vi "NavX Variable Get.vi"(8 "error in":errorcluster) -> ()   [LabVIEW 2017]
uses:
  <vilib>/Rock Robotics/SystemInterfaces/spilib/spi_bus.ctl
  navx-mxp/labview/navX Library v2/IO/Open/Z900_navX_Open_SPI.vi
  navx-mxp/labview/navX Library v2/navX Library v2.lvlib
panel:
  in  "G Force":dbl=3.0
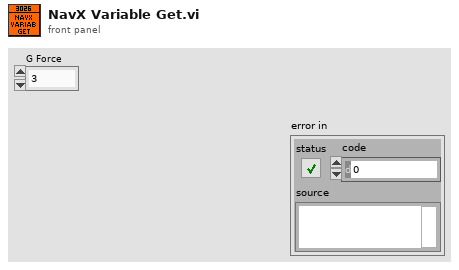
[diagram p1: front panel]
types:
  T1 = typedef "spi_bus.ctl" = enum16{"SPI On-Board, CS0", "SPI On-Board, CS1", "SPI On-Board, CS2", "SPI On-Board, CS3", "SPI MXP", "Invalid"}
  T2 = typedef "navX Library v2.lvlib/Z900_navX_DeviceTypeDef.ctl" = cluster{"Interface":cluster{"Protocol":T3, "Update Rate (4Hz-100Hz)":u8, "navX Open TypeDef":variant}, "Notify Packet":refnum<notifier>, "Loop VI Refnum":refnum<vi>, "Ready to Close Occurrence Refnum":refnum<k4>}
  T3 = typedef "navX Library v2.lvlib/Z900_navX_ProtocolTypeDef.ctl" = enum16{"SERIAL", "I2C", "SPI"}
  T4 = cluster{"Quat W":dbl, "Quat X":dbl, "Quat Y":dbl, "Quat Z":dbl}
  T5 = cluster{"Velocity X":dbl, "Velocity Y":dbl, "Velocity Z":dbl, "Displacement X":dbl, "Displacement Y":dbl, "Displacement Z":dbl}
  T6 = cluster{"Yaw":dbl, "Roll":dbl, "Pitch":dbl, "Heading":dbl, "Fused Heading":dbl}
  T7 = cluster{"LinearAcceleration X":dbl, "LinearAcceleration Y":dbl, "LinearAcceleration Z":dbl}
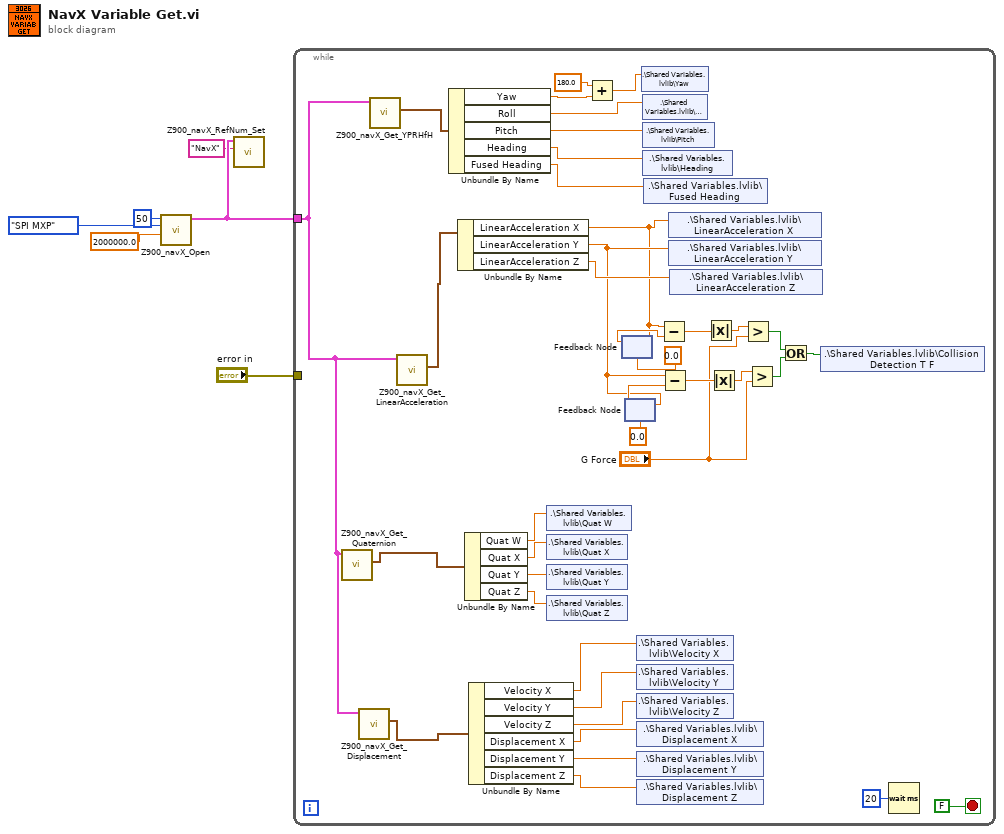
[diagram p0: block diagram]
diagram:
  n1 = call-poly "Z900_navX_Open.vi"("Clock Rate (Hz)"=2000000.0, "SPI Bus"=spi_bus."SPI MXP", "Update Rate (4Hz-60Hz)"=u8 50) -> ("navX Device"=w2:T2)  [unwired: 7 in, 1 out]
  n2 = call "Z900_navX_RefNum_Set.vi"("refnum name"="NavX", "navX Device"=w2) -> ()  [unwired: 8 in, 2 out]
  n3 = while {
    tunnel: "error in" -> [_]
    tunnel: w2 -> [w7]
    stop <- FALSE stop-if-true
    n4 = call "Z900_navX_Get_Quaternion.vi"("navX Device"=w7) -> ("Quaternion"=w9:T4)  [unwired: 7 in, 3 out]
    n5 = call "Z900_navX_Get_Displacement.vi"("navX Device"=w7) -> ("Displacement"=w10:T5)  [unwired: 7 in, 3 out]
    n6 = call "Z900_navX_Get_YPRHfH.vi"("navX Device"=w7) -> ("YRPHfH"=w11:T6)  [unwired: 7 in, 3 out]
    n7 = call "Z900_navX_Get_LinearAcceleration.vi"("navX Device"=w7) -> ("Linear Acceleration"=w8:T7)  [unwired: 7 in, 3 out]
    n8 = Unbundle By Name(w11) -> ("Yaw"=w33:dbl, "Roll"=w27:dbl, "Pitch"=w45:dbl, "Heading"=w44:dbl, "Fused Heading"=w43:dbl)
    n9 = Unbundle By Name(w8) -> ("LinearAcceleration X"=w12:dbl, "LinearAcceleration Y"=w21:dbl, "LinearAcceleration Z"=w42:dbl)
    n10 = Unbundle By Name(w9) -> ("Quat W"=w30:dbl, "Quat X"=w41:dbl, "Quat Y"=w40:dbl, "Quat Z"=w39:dbl)
    n11 = Unbundle By Name(w10) -> ("Velocity X"=w38:dbl, "Velocity Y"=w29:dbl, "Velocity Z"=w37:dbl, "Displacement X"=w36:dbl, "Displacement Y"=w31:dbl, "Displacement Z"=w35:dbl)
    n12 = shared-variable ".\\Shared Variables.lvlib\\Quat W"(w30) -> ()  [unwired: 1 in, 1 out]
    n13 = shared-variable ".\\Shared Variables.lvlib\\Quat X"(w41) -> ()  [unwired: 1 in, 1 out]
    n14 = shared-variable ".\\Shared Variables.lvlib\\Quat Y"(w40) -> ()  [unwired: 1 in, 1 out]
    n15 = shared-variable ".\\Shared Variables.lvlib\\Quat Z"(w39) -> ()  [unwired: 1 in, 1 out]
    n16 = Add(x=180.0, y=w33) -> (x+y=w26:dbl)
    n17 = feedback #1(0.0 ("LinearAcceleration X")) -> (w20:dbl)
    n18 = feedback-in #1(w12) -> ()
    n19 = feedback-in #2(w21) -> ()
    n20 = feedback #2(0.0 ("LinearAcceleration Y")) -> (w22:dbl)
    n21 = shared-variable ".\\Shared Variables.lvlib\\Velocity X"(w38) -> ()  [unwired: 1 in, 1 out]
    n22 = shared-variable ".\\Shared Variables.lvlib\\Velocity Y"(w29) -> ()  [unwired: 1 in, 1 out]
    n23 = shared-variable ".\\Shared Variables.lvlib\\Velocity Z"(w37) -> ()  [unwired: 1 in, 1 out]
    n24 = shared-variable ".\\Shared Variables.lvlib\\Displacement X"(w36) -> ()  [unwired: 1 in, 1 out]
    n25 = shared-variable ".\\Shared Variables.lvlib\\Displacement Y"(w31) -> ()  [unwired: 1 in, 1 out]
    n26 = shared-variable ".\\Shared Variables.lvlib\\Displacement Z"(w35) -> ()  [unwired: 1 in, 1 out]
    n27 = shared-variable ".\\Shared Variables.lvlib\\Yaw"(w26) -> ()  [unwired: 1 in, 1 out]
    n28 = shared-variable ".\\Shared Variables.lvlib\\Roll"(w27) -> ()  [unwired: 1 in, 1 out]
    n29 = shared-variable ".\\Shared Variables.lvlib\\Pitch"(w45) -> ()  [unwired: 1 in, 1 out]
    n30 = shared-variable ".\\Shared Variables.lvlib\\Heading"(w44) -> ()  [unwired: 1 in, 1 out]
    n31 = shared-variable ".\\Shared Variables.lvlib\\Fused Heading"(w43) -> ()  [unwired: 1 in, 1 out]
    n32 = Subtract(x=w12, y=w20) -> (x-y=w25:dbl)
    n33 = Subtract(x=w21, y=w22) -> (x-y=w23:dbl)
    n34 = shared-variable ".\\Shared Variables.lvlib\\LinearAcceleration X"(w12) -> ()  [unwired: 1 in, 1 out]
    n35 = shared-variable ".\\Shared Variables.lvlib\\LinearAcceleration Y"(w21) -> ()  [unwired: 1 in, 1 out]
    n36 = shared-variable ".\\Shared Variables.lvlib\\LinearAcceleration Z"(w42) -> ()  [unwired: 1 in, 1 out]
    n37 = Absolute Value(x=w25) -> (abs(x)=w24:dbl)
    n38 = Absolute Value(x=w23) -> (abs(x)=w14:dbl)
    n39 = Greater?(x=w24, y="G Force") -> (0:w16:bool)
    n40 = Greater?(x=w14, y="G Force") -> (0:w17:bool)
    n41 = Or(x=w16, y=w17) -> (x .or. y?=w15:bool)
    n42 = shared-variable ".\\Shared Variables.lvlib\\Collision Detection T F"(w15) -> ()  [unwired: 1 in, 1 out]
    n43 = Wait (ms)(milliseconds to wait=u32 20) -> ()  [unwired: 1 out]
  }
